vi "CloseAppRefInArray.vi"(1 "Array":refnum<vi>[](array[refnum])) -> (0 "error out":errorcluster)   [LabVIEW 2010]
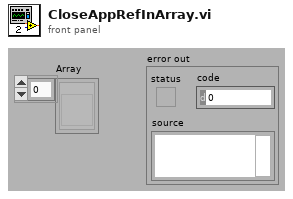
[diagram p1: front panel]
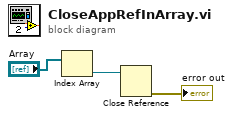
[diagram p0: block diagram]
diagram:
  n1 = Index Array(array="Array") -> (element=w1:refnum<vi>)  [unwired: 1 in]
  n2 = Close Reference(reference=w1) -> (error out=→"error out":errorcluster)  [unwired: 1 in]
